vi "IAmEngine-CreateDVR-ForIAmGLF.vi"(8 "error in (no error)":errorcluster, 9 "IAmGLF Return Notifier":refnum<notifier>, 10 "IAmGLF To Create DVR":refnum<class "IAmGLF.lvclass">, 11 "IAmEngine in":refnum<class "IAmEngine.lvclass">) -> (0 "error out":errorcluster, 3 "IAmEngine out":refnum<class "IAmEngine.lvclass">)   [LabVIEW 2024, in "GLF.lvlib" / "IAmEngine.lvclass"]
doc: "<B>Summary</B>\nCreate DVR for <B>IAmEngine To Create DVR</B>\n\n<B>Details</B>\nThis is really here to reduce coupling between GLF classes. Engine will depend on other classes (Window, View, etc...). But the way I want to use them would require them to depend on Engine too, inducing circular dependency."
uses:
  IAmEngine.lvclass
  IAmGLF/IAmGLF.lvclass
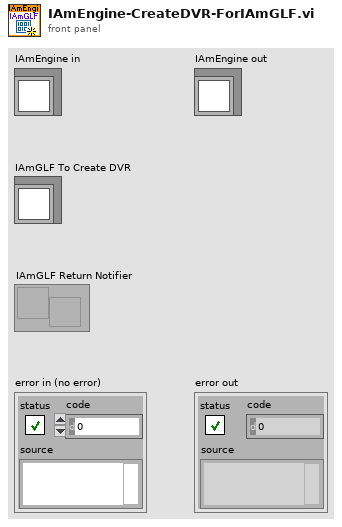
[diagram p1: front panel]
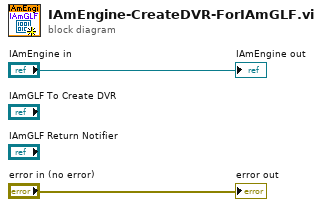
[diagram p0: block diagram]
diagram:
  "error out" <- "error in (no error)"
  "IAmEngine out" <- "IAmEngine in"
